vi "create_waveform_array.vi"(7 "channel info array":cluster{"Module":string, "Channel":string}[](array[cluster]) caption="通道信息数组", 8 "error in (no error)":errorcluster caption="错误输入（无错误）", 9 "samples to write":dbl[][](array[numeric]) caption="待写入采样点", 10 "sampling period (s)":dbl caption="采样周期 (s)", 11 "Timestamp":timestamp caption="时间标识") -> (0 "error out":errorcluster caption="错误输出", 3 "Waveform Array":waveform(dbl)[](array[waveform]) caption="波形数据")   [LabVIEW 2015]
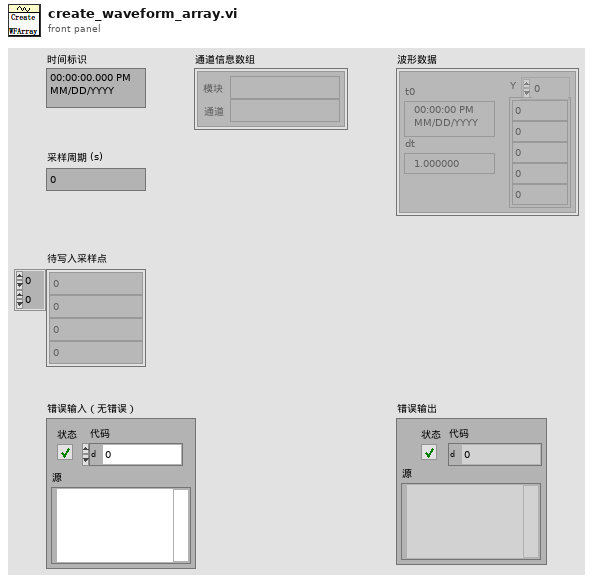
[diagram p1: front panel]
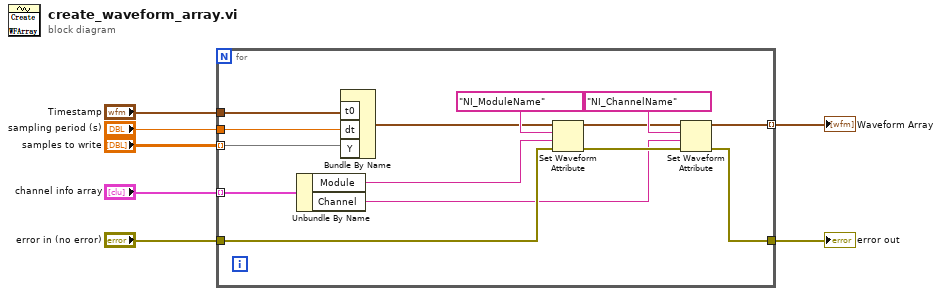
[diagram p0: block diagram]
diagram:
  n1 = for {
    tunnel: [w21] -> w3 mode=indexing
    tunnel: "error in (no error)" -> [w20]
    tunnel: [w18] -> w6
    tunnel: "samples to write" -> [w13] mode=indexing
    tunnel: "Timestamp" -> [w12]
    tunnel: "channel info array" -> [w11] mode=indexing
    tunnel: "sampling period (s)" -> [w8]
    n2 = Unbundle By Name(w11) -> ("Module"=w9:string, "Channel"=w10:string)
    n3 = Bundle By Name("t0"=w12, "dt"=w8, "Y"=w13) -> (w15:waveform(dbl))  [unwired: 1 in]
    n4 = Set Waveform Attribute(4:w20, 5:w9, 6:"NI_ModuleName", 7:w15) -> (0:w19:errorcluster, 3:w14:waveform(dbl))  [unwired: 1 out]
    n5 = Set Waveform Attribute(4:w19, 5:w10, 6:"NI_ChannelName", 7:w14) -> (0:w18:errorcluster, 3:w21:waveform(dbl))  [unwired: 1 out]
  }
  "error out" <- w6
  "Waveform Array" <- w3
